vi "format reuse control and menu.vi"(4 "My Name":T1, 5 "error in (no error)":errorcluster, 6 "Menu Refnum":refnum<k9>, 7 "GUI Refnum in":refnum<vi>, 8 "Save Button":refnum<vi>) -> (0 "error out":errorcluster, 2 "GUI Refnum out":refnum<vi>, 3 "Save Button Out":refnum<vi>)   [LabVIEW 2015, in "Startup Processes.lvlib"]
uses:
  Startup Processes.lvlib
  _typedefs/Subpanel Names.ctl
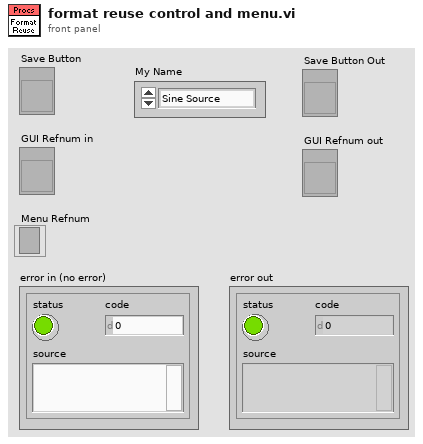
[diagram p1: front panel]
types:
  T1 = typedef "Startup Processes.lvlib/Subpanel Names.ctl" = enum16{"Sine Source", "Ramp Source", "Hen House TC", "Dog House TC", "Out House TC"}
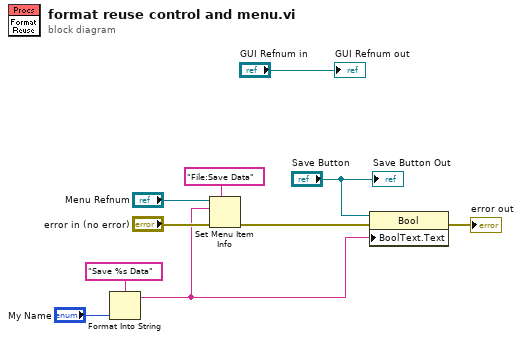
[diagram p0: block diagram]
diagram:
  n1 = Format Into String(format string="Save %s Data", "My Name") -> (resulting string=w2:string)  [unwired: 2 in, 1 out]
  n2 = Set Menu Item Info(7:"File:Save Data" ("item tag"), 8:"error in (no error)", 10:w2, 11:"Menu Refnum") -> (0:w3:errorcluster)  [unwired: 3 in, 1 out]
  n3 = property class="Bool"(reference="Save Button", error in=w3, "BoolText.Text"=w2) -> (error out=→"error out":errorcluster)  [unwired: 1 out]
  "GUI Refnum out" <- "GUI Refnum in"
  "Save Button Out" <- "Save Button"
